vi "onBoard LED single set.vi"(8 "Error In":errorcluster, 9 "new state":bool, 10 "LED index":i32) -> (0 "Error Out":errorcluster)   [LabVIEW 2019]
uses:
  FPGA/FPGA varible.vi
  <vilib>/Utility/error.llb/Error Cluster From Error Code.vi
  <vilib>/rvi/errors/niLvFpgaAdjustHostInterfaceError.vi
  <vilib>/rvi/interface/nirviReadWriteControl/nirviReadWriteControl.xnode
  NiFpgaLv.dll
  <vilib>/rvi/interface/Simulation/niFpgaSimulationCallBeginRW.vi
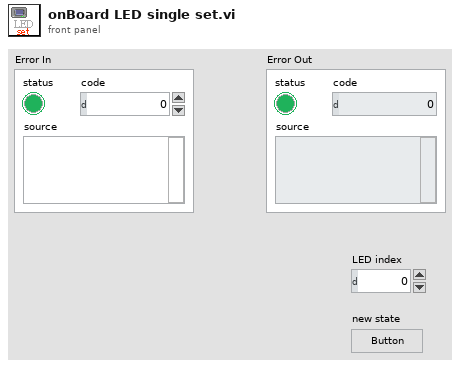
[diagram p1: front panel]
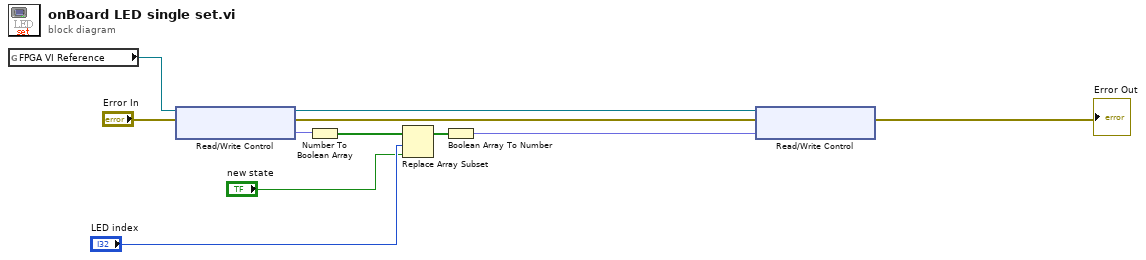
[diagram p0: block diagram]
diagram:
  n1 = global read "FPGA varible.vi" "FPGA VI Reference"() -> (w11:refnum<k20>)
  n2 = xnode "Read/Write Control"("FPGA VI Reference In"=w11, "error in"="Error In") -> ("FPGA VI Reference Out"=w8:refnum<k20>, "error out"=w9:errorcluster, "OnBoard.LED[3:0]"=w7:fxp<+,4,4>)
  n3 = Number To Boolean Array(number=w7) -> (Boolean array=w6:bool[])
  n4 = Replace Array Subset(array=w6, new element="new state", index="LED index") -> (w3:bool[])
  n5 = Boolean Array To Number(Boolean array=w3) -> (number=w2:fxp<+,4,4>)
  n6 = xnode "Read/Write Control"("FPGA VI Reference In"=w8, "error in"=w9, "OnBoard.LED[3:0]"=w2) -> ("error out"=→"Error Out":errorcluster)  [unwired: 1 out]
